vi "subvi1.vi"() -> ()   [LabVIEW 2021]
panel:
  in  "F":dbl
  out "Thermometer":dbl(slide) scale=0.0..100.0
  in  "stop":bool
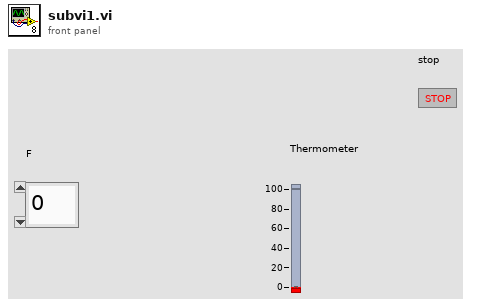
[diagram p1: front panel]
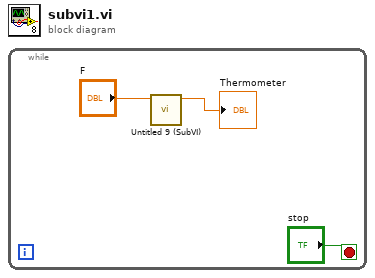
[diagram p0: block diagram]
diagram:
  n1 = while {
    stop <- "stop" stop-if-true
    n2 = call "Untitled 9 (SubVI).vi"("F"="F") -> ("Numeric"=→"Thermometer":dbl)  [unwired: 10 in]
  }
